vi "Creators Creator Queue.vi"(9 "Priority?":bool, 10 "Msg Strategy":refnum<class "Msg Strategy.lvclass">, 11 "Template Event in":refnum<class "Template Event.lvclass">) -> (3 "Template Event out":refnum<class "Template Event.lvclass">)   [LabVIEW 2021, in "Template Event.lvlib" / "Template Event.lvclass"]
uses:
  Template Event.lvclass
  <vilib>/Nathan Davis/jettl/jettl/Msg Strategy/Msg Strategy.lvclass
  Template Event.lvclass/Template Event.ctl
  <vilib>/Nathan Davis/jettl/jettl/Event/Event.lvclass
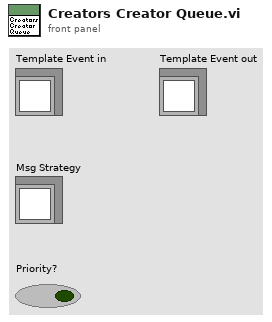
[diagram p1: front panel]
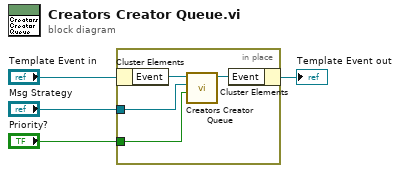
[diagram p0: block diagram]
diagram:
  n1 = in-place {
    in-place-border: "Msg Strategy" -> [w6]
    in-place-border: "Priority?" -> [w5]
    n2 = in-place-cluster #1("Template Event in") -> ("Event"=w8:refnum<class "Event.lvclass">)
    n3 = call-dynamic "Creators Creator Queue.vi"("Priority?"=w5, "Msg Strategy"=w6, "Event in"=w8) -> ("Event out"=w7:refnum<class "Event.lvclass">)  [unwired: 8 in]
    n4 = in-place-cluster #1("Event"=w7) -> (→"Template Event out":refnum<class "Template Event.lvclass">)
  }
